vi "Encode JSON String.vi"(0 "string in":string, 11 "error in (no error)":errorcluster) -> (4 "JSON string out":string, 15 "error out":errorcluster)   [LabVIEW 2020, in "MeasurementLink Measurement Server.lvlib"]
uses:
  MeasurementLink Measurement Server.lvlib
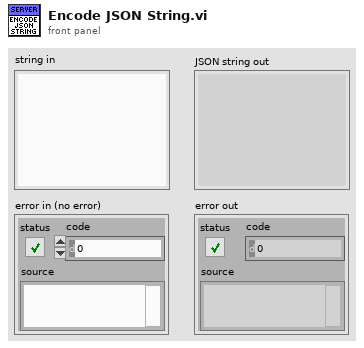
[diagram p1: front panel]
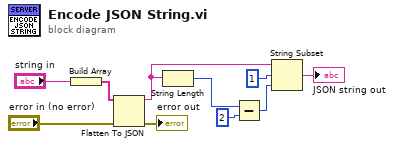
[diagram p0: block diagram]
diagram:
  n1 = Build Array("string in") -> (w10:string[])
  n2 = Flatten To JSON(anything=w10, error in (no error)="error in (no error)") -> (JSON string=w5:string, 11:→"error out":errorcluster)  [unwired: 1 in]
  n3 = String Length(string=w5) -> (length=w9:i32)
  n4 = Subtract(x=w9, y=2) -> (x-y=w7:i32)
  n5 = String Subset(string=w5, offset (0)=1, length (rest)=w7) -> (substring=→"JSON string out":string)
